vi "calibrate.vi"() -> ()   [LabVIEW 2014]
uses:
  <vilib>/userdefined/High Color/IMAQdx.ctl
  <vilib>/vision/driver/NI_Vision_Acquisition_Software.lvlib
  <resource>/objmgr/imaqdx.rc
panel:
  out "Cluster":cluster{"Sensor Width":u32, "Sensor Height":u32}
  in  "Pixel Size in µm":dbl=5.5
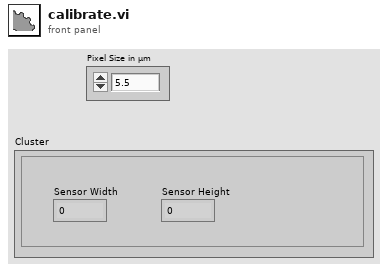
[diagram p1: front panel]
types:
  T1 = typedef "IMAQdx.ctl" = refnum<k21>
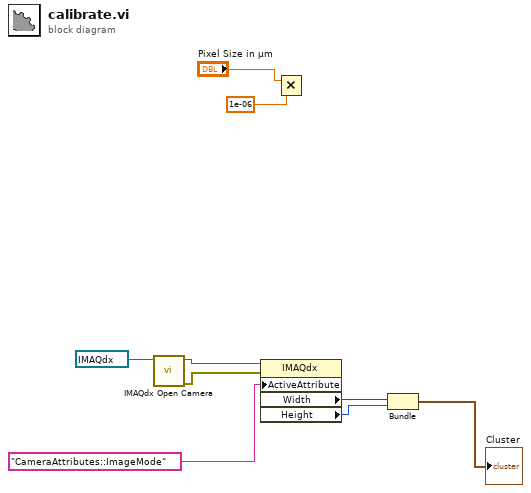
[diagram p0: block diagram]
diagram:
  n1 = call <vilib>:"IMAQdx Open Camera.vi"("Session In"=T1 "cam0") -> ("error out"=w6:errorcluster, "Session Out"=w7:T1)  [unwired: 9 in]
  n2 = property class="IMAQdx"(reference=w7, error in=w6, "ActiveAttribute"="CameraAttributes::ImageMode") -> ("Width"=w3:u32, "Height"=w2:u32)  [unwired: 2 out]
  n3 = Multiply(x="Pixel Size in µm", y=1e-06) -> ()  [unwired: 1 out]
  n4 = Bundle("Width"=w3, "Height"=w2) -> (→"Cluster":cluster{"Width":u32, "Height":u32})  [unwired: 1 in]
